vi "Message Listener.vi"(0 "Vision Server":T1, 1 "error in":errorcluster) -> (2 "Vision Server":T1, 3 "Vision Update":T2, 4 "error out":errorcluster)   [LabVIEW 2016]
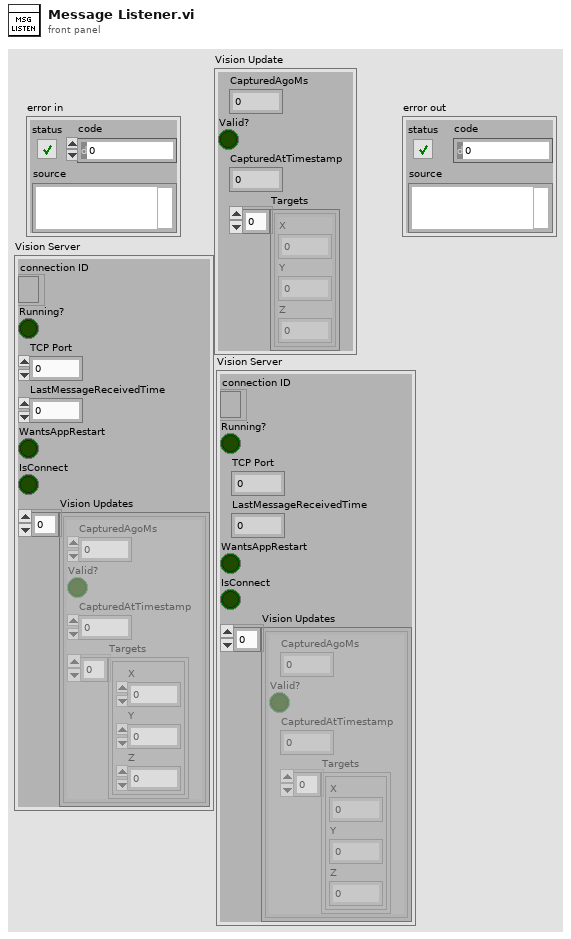
[diagram p1: front panel]
types:
  T1 = cluster{"connection ID":refnum<k5>, "Running?":bool, "TCP Port":u16, "LastMessageReceivedTime":dbl, "WantsAppRestart":bool, "IsConnect":bool, "Vision Updates":cluster{"CapturedAgoMs":i32, "Valid?":bool, "CapturedAtTimestamp":dbl, "Targets":cluster{"X":dbl, "Y":dbl, "Z":dbl}[]}[]}
  T2 = cluster{"CapturedAgoMs":i32, "Valid?":bool, "CapturedAtTimestamp":dbl, "Targets":cluster{"X":dbl, "Y":dbl, "Z":dbl}[]}
  T3 = enum16{"Standard", "Buffered", "CRLF", "Immediate"}
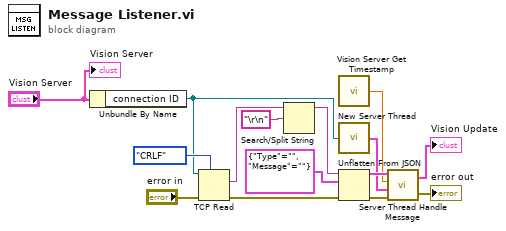
[diagram p0: block diagram]
diagram:
  n1 = Unbundle By Name("Vision Server") -> ("connection ID"=w9:refnum<k5>)
  n2 = TCP Read(connection ID=w9, error in (no error)="error in", 7:T3."CRLF" ("mode (standard)")) -> (data out=w14:string, error out=w5:errorcluster)  [unwired: 2 in, 1 out]
  n3 = Search/Split String(string=w14, search string/char (-)="\r\n") -> (substring before match=w12:string)  [unwired: 1 in, 2 out]
  n4 = call "Vision Server Get Timestamp.vi"() -> ("Timestamp (ms)"=w7:dbl)
  n5 = call "New Server Thread.vi"("connection ID"=w9) -> ("Server Thread"=w8:cluster{"connection ID":refnum<k5>})
  n6 = Unflatten From JSON(JSON string=w12, type and defaults=cluster{"Type":string, "Message":string} {"Type"="", "Message"=""} ("input cluster"), error in (no error)=w5) -> (value=w10:cluster{"Type":string, "Message":string}, error out=w6:errorcluster)  [unwired: 4 in]
  n7 = call "Server Thread Handle Message.vi"("error in"=w6, "Server Thread"=w8, "Timestamp"=w7, "Vision Message"=w10) -> ("error out"=→"error out":errorcluster, "Vision Update"=→"Vision Update":T2)
  "Vision Server" <- "Vision Server"
